vi "Util-Report Instr. Specific Error.vi"(7 "source":string, 8 "error in (no error)":errorcluster, 9 "error message":string, 10 "new error":bool, 11 "VISA resource name":refnum<visa-resource-name>) -> (0 "error out":errorcluster, 3 "VISA resource name out":refnum<visa-resource-name>)   [LabVIEW 2016, in "Agilent 415X Series.lvlib"]
doc: "This is a utility VI which reports instrument specific errors when:\n - new error is set to TRUE (ie. there is a new error present)\n - no previous error (no error in \"Error In\" is TRUE).\nso that only the first error occurred will be reported.\n\nThen \n - \"no error\" in \"Error Out\" will be set to \"FALSE\"\n - \"code\" will be set to \"-1300\" - instrument specific error.\n - \"source\" will be set to \"source\" and \"error message\"."
uses:
  Agilent 415X Series.lvlib
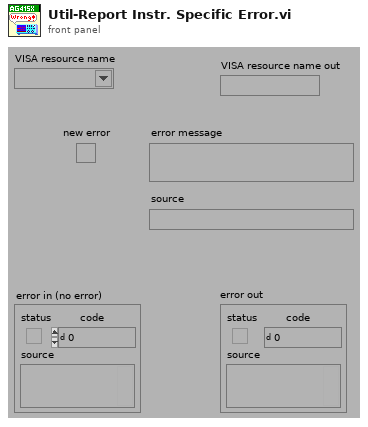
[diagram p1: front panel]
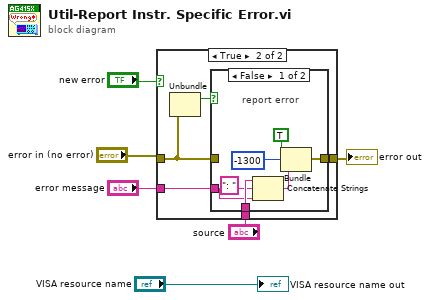
[diagram p0: block diagram]
diagram:
  n1 = case shown="True" "new error" {
    tunnel: [w7 w10] -> w3
    tunnel: "error in (no error)" -> [w7 w11]
    tunnel: "error message" -> [_ w9]
    tunnel: "source" -> [_ w8]
    frame False {
      # "no new error"
    }
    frame True {
      n2 = Unbundle(w11) -> ("status"=w12:bool)  [unwired: 2 out]
      n3 = case shown="False" w12 {
        tunnel: w11 -> [_ w20]
        tunnel: [w17 w20] -> w10
        tunnel: w9 -> [w14 _]
        tunnel: w8 -> [w15 _]
        frame False {
          # "report error"
          n4 = Concatenate Strings(w15, ": ", w14) -> (w16:string)
          n5 = Bundle(TRUE, -1300, w16) -> (w17:errorcluster)  [unwired: 1 in]
        }
        frame True {
          # "previous error\nexisting"
        }
      }
    }
  }
  "error out" <- w3
  "VISA resource name out" <- "VISA resource name"
